vi "Meas Result Generate TWM Digitizer Correction.vi"(8 "error in":errorcluster, 11 "meas":T4={"swp cfg"={"N"=0, "R"=0, "f list"=[], "smpl delay"=0.0, "set delay"=0.0, "set delay np"=0.0, "meas root"=path "", "meas name"="", "meas a-index"=FALSE, "rnd sweep"=FALSE, "mode"=enum."Frequency", "swp mode"=enum."Linear", "avg"=0, "subrec"=0, "multi-freq"=FALSE}, "bridge"={"type"=enum."TWM client", "TWM"={"pipe name"="", "parameters"=[], "handle"=0, "fixed aper [s]"=0.0, "f-list [Hz]"=[], "discrete f-list"=FALSE, "unc mode"=enum."None", "unc mcc"=0, "unc first"=FALSE}, "last f"=0.0, "bias comp"={"bias type"=enum."dummy", "VISA"="", "Enable"=FALSE, "channel qu"=[], "channel Uinit"=[]}, "sim mode"=enum."Generic RLC network", "channel idns"=[], "sim phases"=1}, "src"={"type"=enum."Tektronix AFG3101C", "afg"={"VISA"="", "const"=0.0, "gen DC"=FALSE, "ext ref"=FALSE}, "cDAQ dds"={"device"="", "channels"=[], "mclk source"="", "mclk [Hz]"=0.0, "use ext mclk"=FALSE, "fs [Hz]"=0.0, "block [s]"=0.0, "buf [s]"=0.0, "task"="", "cmd queue"=refnum, "proc ref"=refnum, "smpl clock out"="/cDAQ3/PFI0", "export smpl clock"=FALSE, "DC ofs [V]"=[]}, "gain [V/A]"=1.0, "F5xxx session"={"VISA"="", "mode"=enum."AC voltage", "Earth on"=FALSE, "Ext ref lock"=FALSE}}, "results"=refnum} {"src"."cDAQ dds"."channels" min=0 step=1; "bridge"."TWM"."f-list [Hz]" format="%#_6p"; "swp cfg"."f list"."bias" format="%#_3p"; "swp cfg"."f list"."level" format="%#_3p"; "swp cfg"."f list"."fs [Hz]" format="%#_5p"; "swp cfg"."f list"."time [s]" format="%#_3p"; "swp cfg"."f list"."f/fs" format="%#_3p"; "swp cfg"."f list"."periods" format="%#_3f"; "swp cfg"."f list"."f [Hz]" format="%#_5p"}) -> (0 "error out":errorcluster)   [LabVIEW 2013]
doc: "Generates simple TWM digitizer correction from measured data."
uses:
  meas session.ctl
  Meas Sweep Config.ctl
  Meas Freq Info.ctl
  meas_swp_mode.ctl
  meas_sweep_flist_mode.ctl
  bridge/Bridge Session.ctl
  bridge/Bridge Type.ctl
  drivers/TWM client/TWM Session.ctl
  drivers/TWM client/TWM parameters.ctl
  drivers/TWM client/Meas Proc QWTB Uncertainty Mode.ctl
  bridge/Bridge Bias Session.ctl
  bridge/Bridge Bias Type.ctl
  bridge/Bridge Sim Mode.ctl
  source/Source Session.ctl
  source/Source Type.ctl
  drivers/AFG3101C/AFG3101C Session.ctl
  drivers/cDAQ DDS/cDAQ DDS Session.ctl
  drivers/cDAQ DDS/cDAQ DDS Setup.ctl
  drivers/Fluke 5XXX/top_lev/F5xxx_session.ctl
  drivers/Fluke 5XXX/top_lev/F5xxx_output_mode.ctl
  Meas Results Ref.ctl
  Meas Results.ctl
  bridge/Bridge Frequency Readings Data.ctl
  drivers/TWM client/Meas Proc QWTB Spectrum Data.ctl
  drivers/TWM client/TWM Phase Info.ctl
  Meas Results Correction Structuring Mode.ctl
  Meas Results TWM Digitizer Correction Data.ctl
  Meas Results TWM Correction Digitizer Type.ctl
panel:
  in  "Digitizer type":T1=enum."HP3458A"
  in  "Estimate non-linearity":bool
  in  "btn exit":bool
  out "last path":path
  out "correction data":T2
  in  "Use aperture correction":bool=TRUE
  in  "Use time shift":bool=TRUE
  in  "Mode":T3
  in  "btn export":bool
  out "table":string[][](table) caption="Overview"
  # "Uncertainty:"
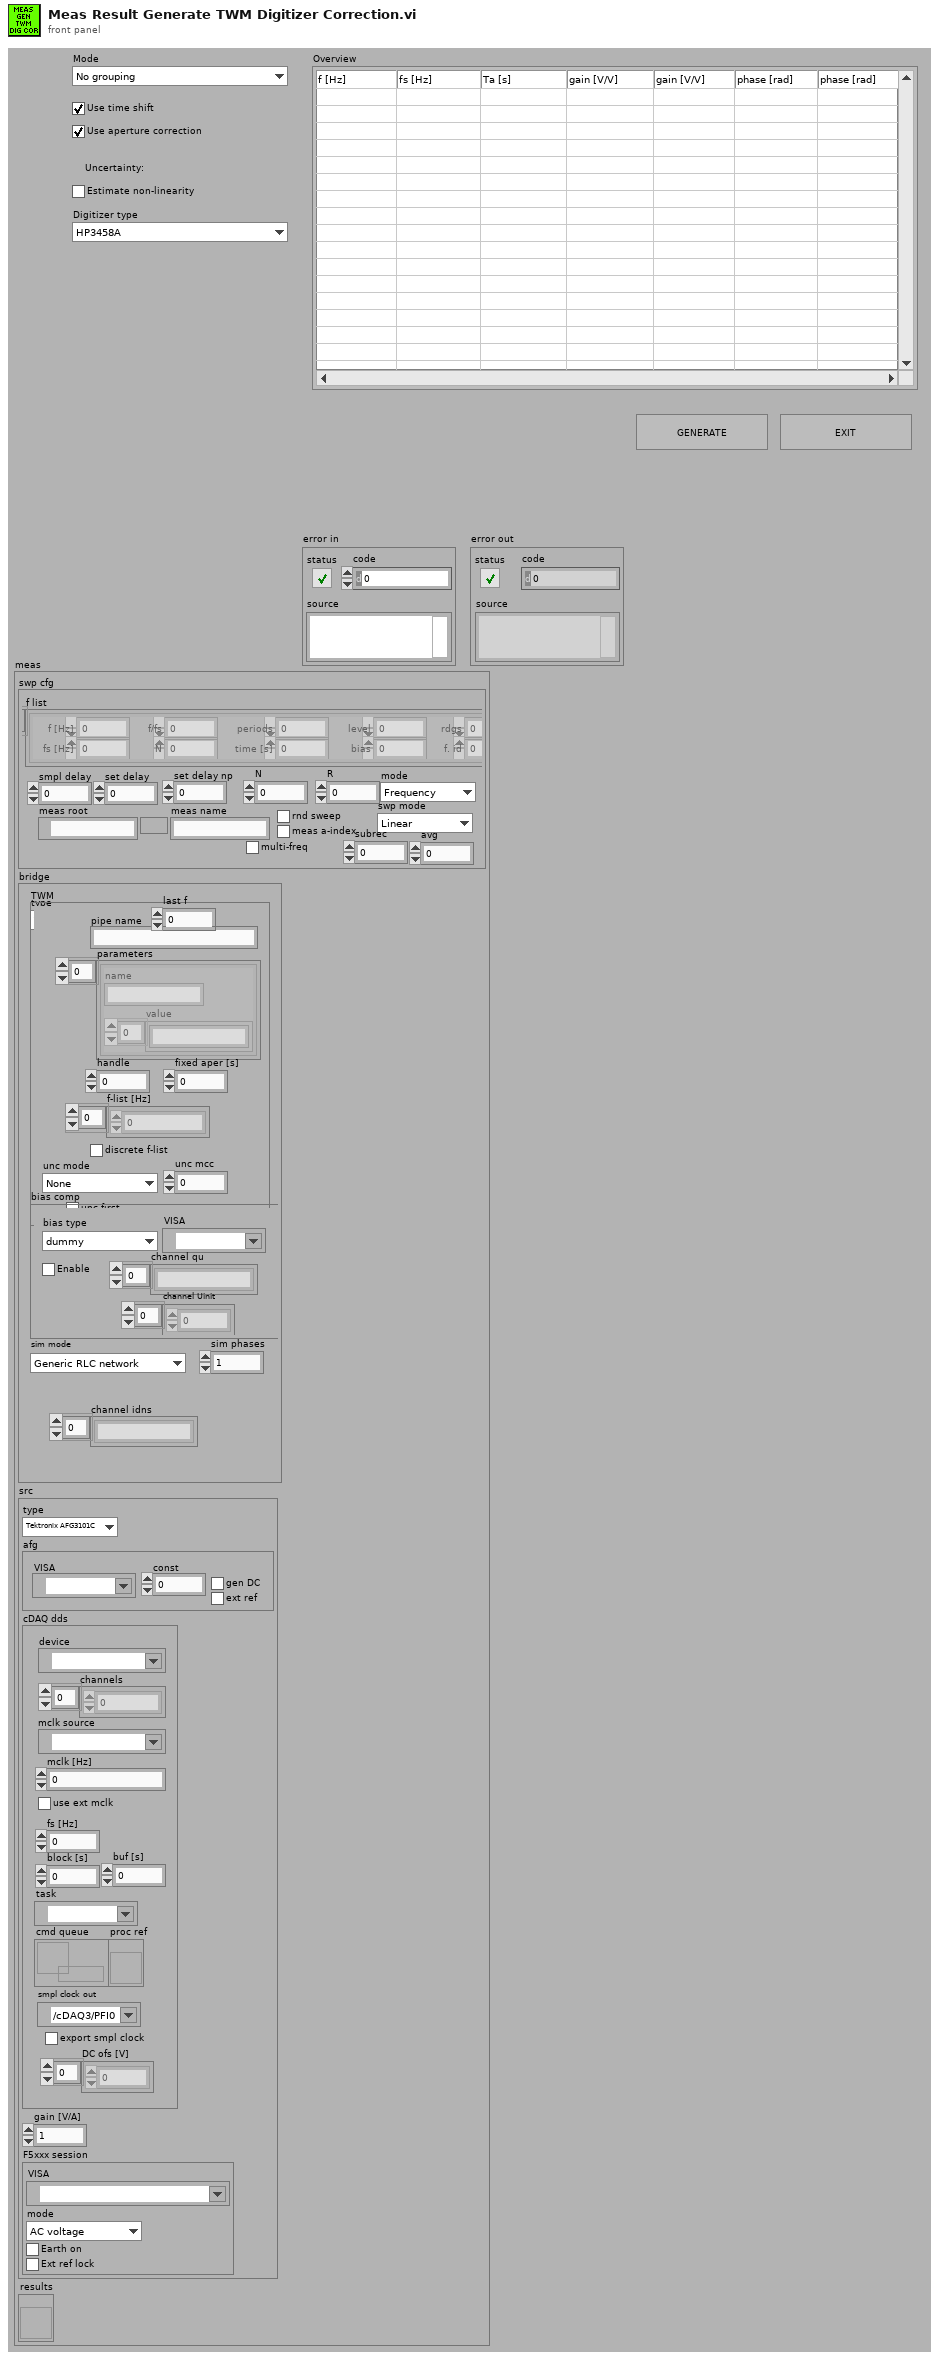
[diagram p1: front panel]
types:
  T1 = typedef "Meas Results TWM Correction Digitizer Type.ctl" = enum16{"Unknown", "HP3458A", "NI9238"}
  T2 = typedef "Meas Results TWM Digitizer Correction Data.ctl" = cluster{"gains [V/V]":dbl[][][], "phases [rad]":dbl[][][], "timeshifts [s]":dbl[][], "f [Hz]":dbl[], "fs list [Hz]":dbl[], "aperture list [s]":dbl[], "channels":string[], "Mode":T3, "aperture correction":bool, "ranges [V]":dbl[], "amp [V]":dbl[][], "apertures [s]":dbl[], "unc gains [V/V]":dbl[][][], "unc phases [rad]":dbl[][][]}
  T3 = typedef "Meas Results Correction Structuring Mode.ctl" = enum16{"No grouping", "Group by apertures (3458A)", "Group by fs (generic digitizer)"}
  T4 = typedef "meas session.ctl" = cluster{"swp cfg":T5, "bridge":T9, "src":T17, "results":T23}
  T5 = typedef "Meas Sweep Config.ctl" = cluster{"N":i32, "R":i32, "f list":T6[], "smpl delay":dbl, "set delay":dbl, "set delay np":dbl, "meas root":path, "meas name":string, "meas a-index":bool, "rnd sweep":bool, "mode":T7, "swp mode":T8, "avg":i32, "subrec":i32, "multi-freq":bool}
  T6 = typedef "Meas Freq Info.ctl" = cluster{"f [Hz]":dbl, "periods":dbl, "f/fs":dbl, "time [s]":dbl, "fs [Hz]":dbl, "N":i32, "level":dbl, "bias":dbl, "rdgs":i32, "f. id":i32}
  T7 = typedef "meas_swp_mode.ctl" = enum16{"Frequency", "Level", "Bias"}
  T8 = typedef "meas_sweep_flist_mode.ctl" = enum16{"Linear", "Log10"}
  T9 = typedef "Bridge Session.ctl" = cluster{"type":T10, "TWM":T11, "last f":dbl, "bias comp":T14, "sim mode":T16, "channel idns":string[], "sim phases":i32}
  T10 = typedef "Bridge Type.ctl" = enum16{"TWM client", "dummy"}
  T11 = typedef "TWM Session.ctl" = cluster{"pipe name":string, "parameters":T12[], "handle":i32, "fixed aper [s]":dbl, "f-list [Hz]":dbl[], "discrete f-list":bool, "unc mode":T13, "unc mcc":i32, "unc first":bool}
  T12 = typedef "TWM parameters.ctl" = cluster{"name":string, "value":string[]}
  T13 = typedef "Meas Proc QWTB Uncertainty Mode.ctl" = enum16{"None", "GUF", "Monte Carlo"}
  T14 = typedef "Bridge Bias Session.ctl" = cluster{"bias type":T15, "VISA":refnum<visa-resource-name>, "Enable":bool, "channel qu":string[], "channel Uinit":dbl[]}
  T15 = typedef "Bridge Bias Type.ctl" = enum16{"dummy", "CMI LiBbias V1.0"}
  T16 = typedef "Bridge Sim Mode.ctl" = enum16{"Generic RLC network", "Interchannel transfer"}
  T17 = typedef "Source Session.ctl" = cluster{"type":T18, "afg":T19, "cDAQ dds":T20, "gain [V/A]":dbl, "F5xxx session":T21}
  T18 = typedef "Source Type.ctl" = enum16{"Tektronix AFG3101C", "cDAQ DAC", "Fluke 5xxx", "Agilent 33120A", "dummy"}
  T19 = typedef "AFG3101C Session.ctl" = cluster{"VISA":refnum<visa-resource-name>, "const":dbl, "gen DC":bool, "ext ref":bool}
  T20 = typedef "cDAQ DDS Session.ctl" = cluster{"device":tag, "channels":i32[], "mclk source":tag, "mclk [Hz]":dbl, "use ext mclk":bool, "fs [Hz]":dbl, "block [s]":dbl, "buf [s]":dbl, "task":refnum<k21>, "cmd queue":refnum<queue>, "proc ref":refnum<vi>, "smpl clock out":tag, "export smpl clock":bool, "DC ofs [V]":dbl[]}
  T21 = typedef "F5xxx_session.ctl" = cluster{"VISA":refnum<visa-resource-name>, "mode":T22, "Earth on":bool, "Ext ref lock":bool}
  T22 = typedef "F5xxx_output_mode.ctl" = enum16{"AC voltage", "AC current"}
  T23 = typedef "Meas Results Ref.ctl" = refnum<vi>
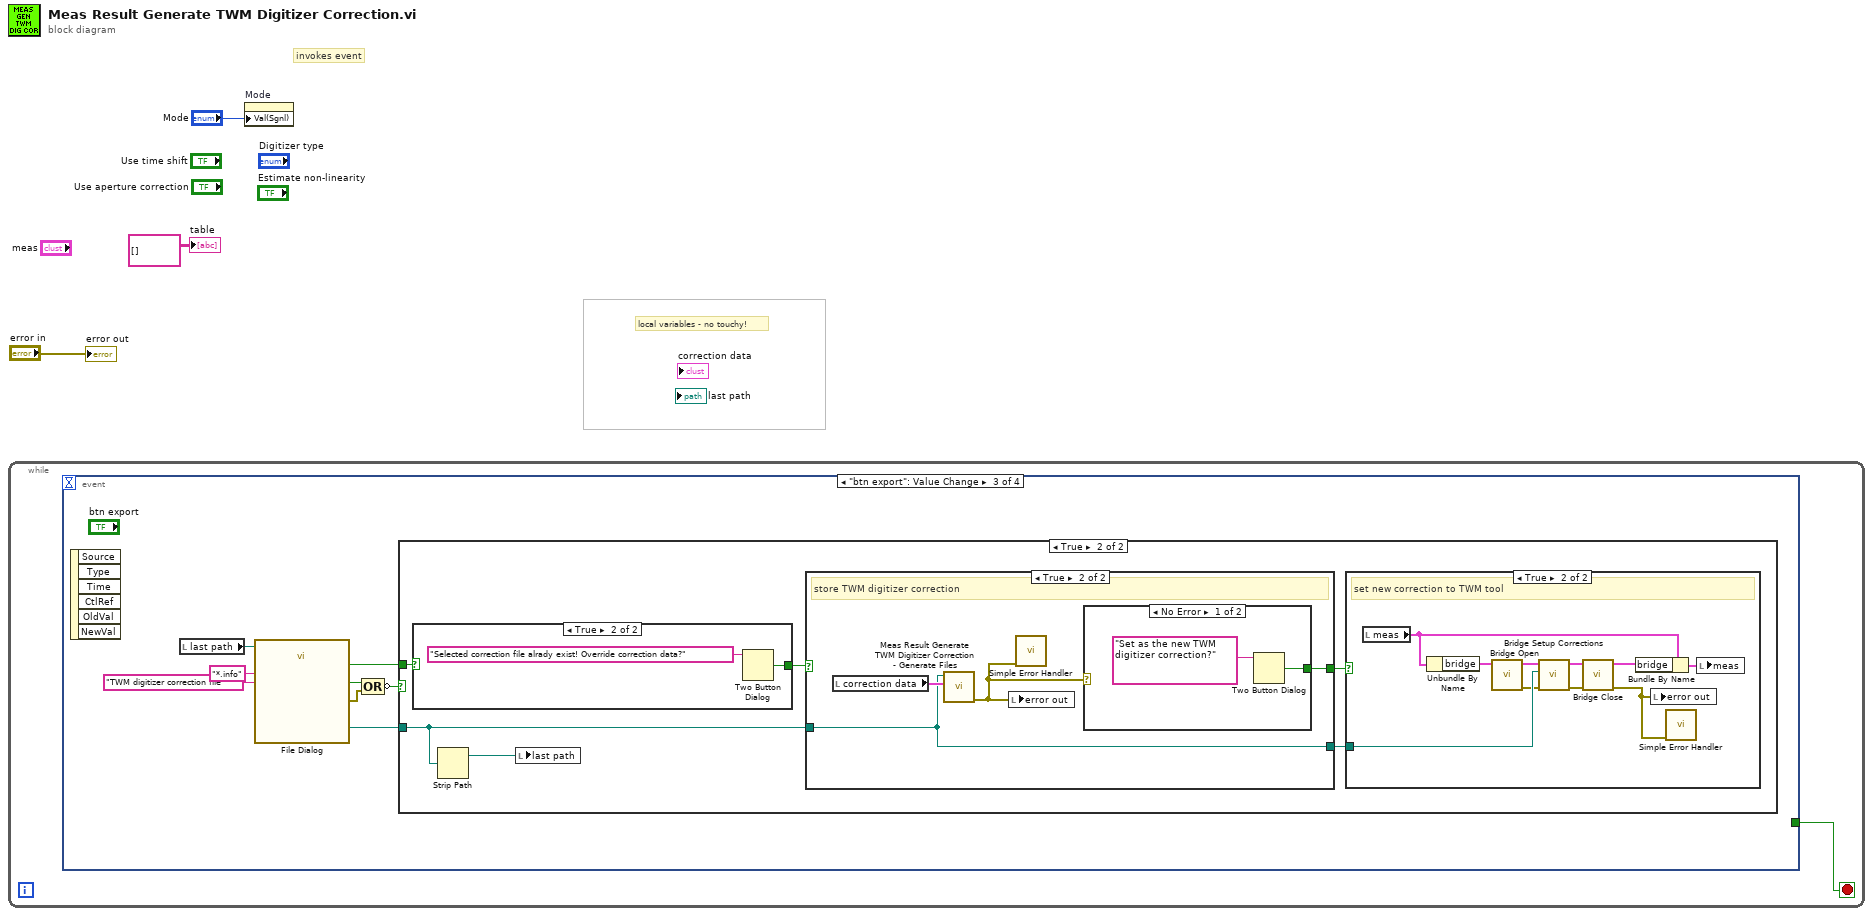
[diagram p0: block diagram]
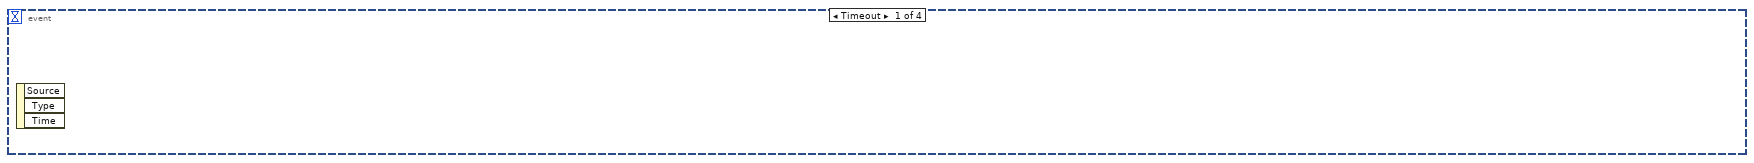
[diagram p2: hidden frame]
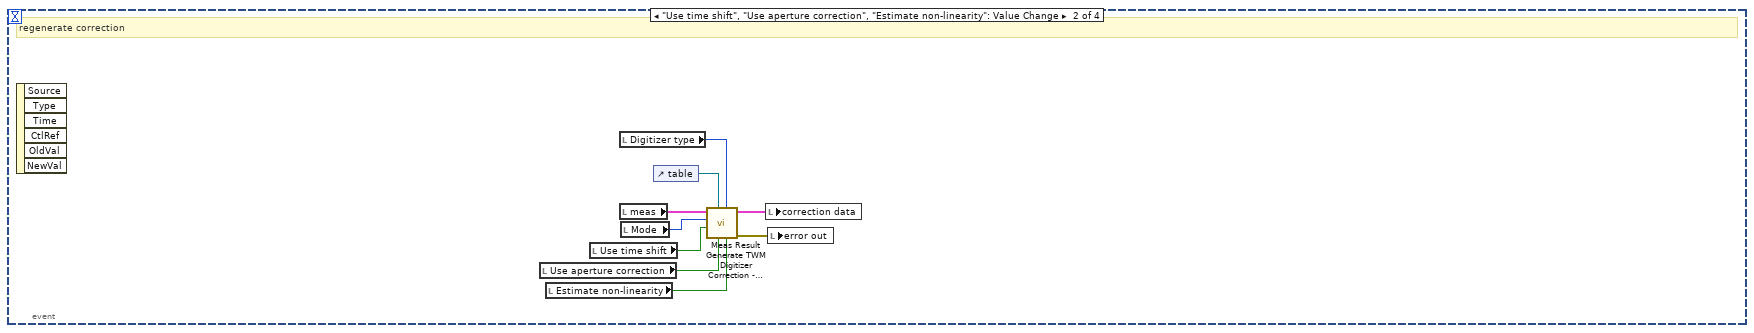
[diagram p3: hidden frame]
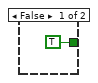
[diagram p6: hidden frame]
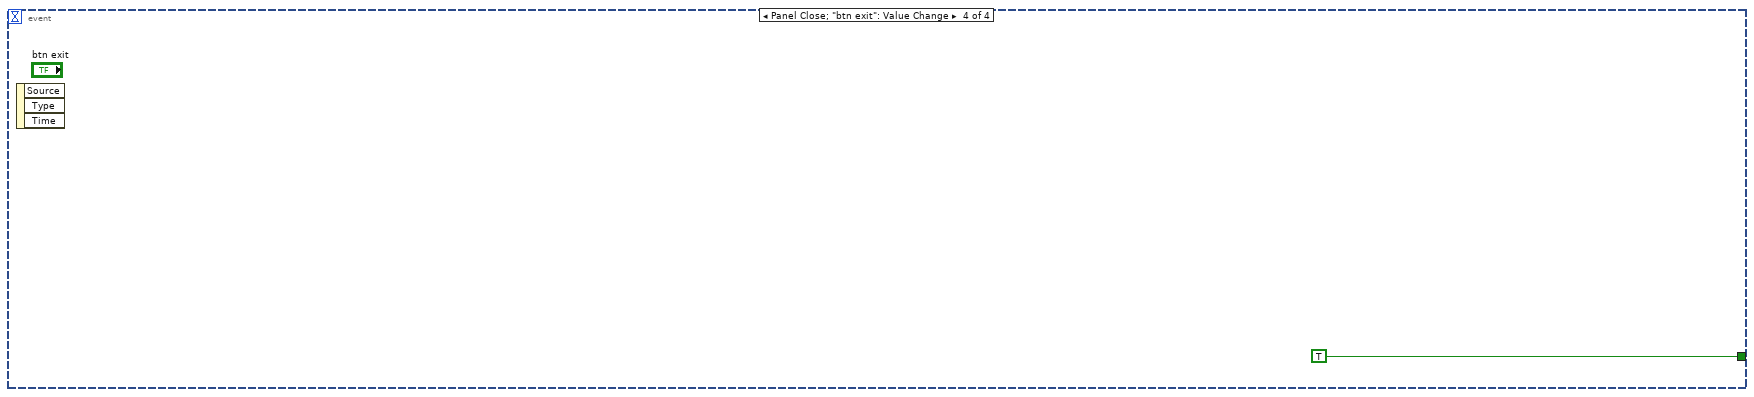
[diagram p9: hidden frame]
diagram:
  # "local variables - no touchy!"
  # "invokes event"
  n1 = while {
    stop <- w4 stop-if-true
    n2 = event shown="[2] \"btn export\": Value Change" {
      selector: _ -> [_ _ _ _]
      dyn-events: _ -> [_ _ _ _]
      timeout: _ -> [_ _ _ _]
      tunnel: [_ _ _ TRUE] -> w4
      event Timeout {
        n3 = event-data() -> ()  [unwired: 1 in, 3 out]
      }
      event "Use time shift", "Use aperture correction", "Estimate non-linearity": Value Change {
        # "regenerate correction"
        n4 = event-data() -> ()  [unwired: 1 in, 6 out]
        n5 = local read "Use aperture correction"() -> (w8:bool)
        n6 = local read "Estimate non-linearity"() -> (w6:bool)
        n7 = local read "Use time shift"() -> (w9:bool)
        n8 = local read "Digitizer type"() -> (w5:T1)
        n9 = local read "meas"() -> (w11:T4)
        n10 = local read "Mode"() -> (w10:T3)
        n11 = control-ref of="table"() -> (w12:refnum<vi>)
        n12 = call "Meas Result Generate TWM Digitizer Correction - Process Measurement.vi"("Estimate non-linearity (False)"=w6, "digitizer type"=w5, "use aperture correction (true)"=w8, "table ref"=w12, "use time shift (true)"=w9, "Mode"=w10, "meas"=w11) -> ("error out"=w13:errorcluster, "correction data"=w7:T2)  [unwired: 3 in]
        n13 = local write "correction data"(w7) -> ()
        n14 = local write "error out"(w13) -> ()
      }
      event "btn export": Value Change {
        n15 = event-data() -> ()  [unwired: 1 in, 6 out]
        n16 = local read "last path"() -> (w14:path)
        n17 = call "File Dialog"("start path"=w14, "pattern (all files)"="*.info", "pattern label"="TWM digitizer correction file") -> ("selected path"=w16:path, "exists"=w15:bool, "cancelled"=w19:bool, "error out"=w18:errorcluster)  [unwired: 9 in]
        n18 = Compound Arithmetic op=OR(w19, w18) -> (invert w17:bool)
        n19 = case shown="True" w17 {
          tunnel: w16 -> [_ w25]
          tunnel: w15 -> [_ w26]
          frame False {
          }
          frame True {
            n20 = case shown="True" w26 {
              tunnel: [TRUE ("T button?") w39] -> w27
              frame False {
              }
              frame True {
                n21 = Two Button Dialog(message="Selected correction file alrady exist! Override correction data?") -> (T button?=w39:bool)  [unwired: 2 in]
              }
            }
            n22 = Strip Path(path=w25) -> (stripped path=w24:path)  [unwired: 1 out]
            n23 = local write "last path"(w24) -> ()
            n24 = case shown="True" w27 {
              tunnel: w25 -> [_ w41]
              tunnel: [_ w42] -> w23
              tunnel: [_ w41] -> w22
              frame False {
              }
              frame True {
                # "store TWM digitizer correction"
                n25 = local read "correction data"() -> (w44:T2)
                n26 = call "Meas Result Generate TWM Digitizer Correction - Generate Files.vi"("correction data"=w44, "correction root file"=w41) -> ("error out"=w43:errorcluster)  [unwired: 9 in]
                n27 = local write "error out"(w43) -> ()
                n28 = call <vilib>:"Simple Error Handler.vi"("error in (no error)"=w43) -> ()  [unwired: 4 in, 5 out]
                n29 = case shown="No Error" w43 {
                  tunnel: [w45 _] -> w42
                  frame No Error {
                    n30 = Two Button Dialog(message="Set as the new TWM digitizer correction?") -> (T button?=w45:bool)  [unwired: 2 in]
                  }
                  frame Error {
                  }
                }
              }
            }
            n31 = case shown="True" w23 {
              tunnel: w22 -> [_ w35]
              frame False {
              }
              frame True {
                # "set new correction to TWM tool"
                n32 = local read "meas"() -> (w37:T4)
                n33 = Unbundle By Name(w37) -> ("bridge"=w34:T9)
                n34 = call "Bridge Open.vi"("bridge in"=w34) -> ("error out"=w32:errorcluster, "bridge out"=w33:T9)  [unwired: 7 in, 2 out]
                n35 = call "Bridge Setup Corrections.vi"("error in"=w32, "digitizer correction path"=w35, "bridge in"=w33) -> ("error out"=w31:errorcluster, "bridge out"=w30:T9)  [unwired: 7 in]
                n36 = call "Bridge Close.vi"("error in"=w31, "bridge in"=w30) -> ("error out"=w28:errorcluster, "bridge out"=w29:T9)  [unwired: 8 in]
                n37 = Bundle By Name(cluster=w37, "bridge"=w29) -> (w36:T4)
                n38 = local write "error out"(w28) -> ()
                n39 = call <vilib>:"Simple Error Handler.vi"("error in (no error)"=w28) -> ()  [unwired: 4 in, 5 out]
                n40 = local write "meas"(w36) -> ()
              }
            }
          }
        }
      }
      event Panel Close; "btn exit": Value Change {
        n41 = event-data() -> ()  [unwired: 1 in, 3 out]
      }
    }
  }
  n42 = property on="Mode" class="Enum (strict)"("Val(Sgnl)"="Mode") -> ()  [unwired: 2 in, 2 out]
  "error out" <- "error in"
  "table" <- string[][] [] ("table")
